vi "Is Homed.vi"(8 "error in (no error)":errorcluster, 11 "Gantry in":refnum<class "Gantry.lvclass">) -> (0 "error out":errorcluster, 2 "homed?":bool, 3 "Gantry out":refnum<class "Gantry.lvclass">)   [LabVIEW 2026, in "Gantry.lvclass"]
uses:
  Gantry.lvclass
  <instrlib>/Aerotech Automation1/Status/TypeDefs/Axis Status Items Cluster.ctl
  <instrlib>/Aerotech Automation1/Status/TypeDefs/Axis Status Item.ctl
  <instrlib>/Aerotech Automation1/Status/Wrappers/Add Axis Status Item.vi
  <instrlib>/Aerotech Automation1/Status/Wrappers/Read Axis Status Item.vi
  <instrlib>/Aerotech Automation1/Status/Status.lvlib
  <instrlib>/Aerotech Automation1/Aerotech Automation1.lvlib
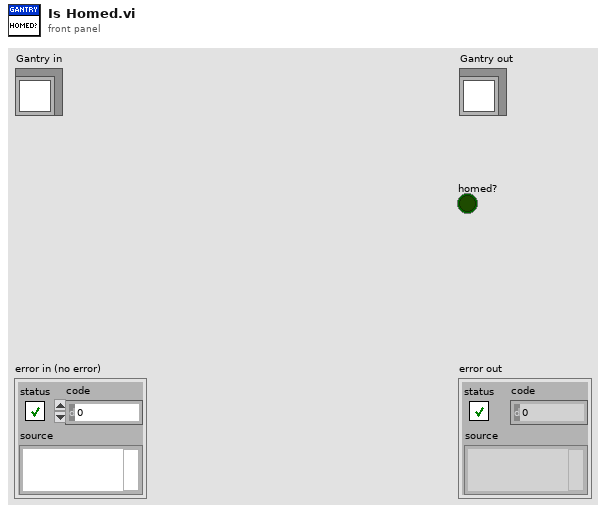
[diagram p1: front panel]
types:
  T1 = typedef "Virtual Modes.ctl" = enum16{"Nonvirtual", "Virtual"}
  T2 = typedef "ControllerDiagPacket.ctl" = cluster{"Number of Diag Packets":i32, "Axes":T3[], "error":errorcluster}
  T3 = typedef "AxisDiagPacket.ctl" = cluster{"Axis Name":string, "Analog Input 0":dbl, "Analog Input 1":dbl, "Axis Fault (num)":i32, "Axis Fault (str)":string, "Axis Fault (bits)":cluster{"AmplifierFault":bool, "AmplifierTemperatureFault":bool, "CcwEndOfTravelLimitFault":bool, "CcwSoftwareLimitFault":bool, "CommunicationLostFault":bool, "CwEndOfTravelLimitFault":bool, "CwSoftwareLimitFault":bool, "EmergencyStopFault":bool, "EncoderFault":bool, "ExternalFault":bool, "FeedbackScalingFault":bool, "GantryMisalignFault ":bool, "HallSensorFault":bool, "InPositionTimeoutFault":bool, "InternalFault":bool, "MarkerSearchFault":bool, "MaxVelocityCommandFault":bool, "MissedInterruptFault":bool, "MotorTemperatureFault":bool, "None":bool, "OverCurrentFault":bool, "PositionErrorFault":bool, "PositionFeedbackFault":bool, "PowerSupplyFault":bool, "ProbeInputFault":bool, "SafeZoneFault":bool, "VelocityErrorFault":bool, "VelocityFeedbackFault":bool, "VoltageClampFault":bool}, "Axis Status (num)":i32, "Axis Status (str)":string, "Axis Status (bits)":cluster{"BacklashActive":bool, "CalibrationEnabled1D":bool, "CalibrationEnabled2D":bool, "CommandValid":bool, "DriveAbortPending":bool, "DrivePending":bool, "Enabling":bool, "GainMappingEnabled":bool, "GantryAligned":bool, "GantryRealigning":bool, "Homed":bool, "Homing":bool, "IFOVEnabled":bool, "JogGenerating":bool, "Jogging":bool, "JoystickControl":bool, "MasterSlaveControl":bool, "MotionBlocked":bool, "MotionClamped":bool, "MoveDone":bool, "None":bool, "NotVirtual":bool, "Profiling":bool, "Stability0":bool, "Stability1":bool, "TrajectoryFiltering":bool, "WaitDone":bool}, "Current Command":sgl, "Current Error":sgl, "Current Feedback":sgl, "Digital Inputs":i32, "Digital Outputs":i32, "Drive Status":i32, "Drive Status (str)":string, "Drive Status (bits)":cluster{"AccelerationPhase":bool, "AutofocusActive":bool, "BrakeOutput":bool, "CcwEndOfTravelLimitInput":bool, "CosineEncoderError":bool, "CurrentClamp":bool, "CwEndOfTravelLimitInput":bool, "DecelerationPhase":bool, "DualLoopActive":bool, "EmergencyStopInput":bool, "Enabled":bool, "EncoderClipping":bool, "GalvoCalibrationEnabled":bool, "GalvoPowerCorrection":bool, "HallAInput":bool, "HallBInput":bool, "HallCInput":bool, "HighResolutionMode":bool, "HomeLimitInput":bool, "InPosition":bool, "InPosition2":bool, "MarkerInput":bool, "MarkerLatch":bool, "MoveActive":bool, "NoMotorSupply":bool, "None":bool, "PowerLimiting":bool, "ProgrammingFlash":bool, "ProgrammingMXH":bool, "PSOHaltLatch":bool, "ServoControl":bool, "SineEncoderError":bool}, "Position Feedback Auxiliary":dbl, "Position Command":dbl, "Position Error":dbl, "Position Feedback":dbl, "Program Position Command":dbl, "Program Position Error":dbl, "Program Position Feedback":dbl, "Velocity Command":dbl, "Velocity Error":dbl, "Velocity Feedback":dbl}
  T4 = typedef "Aerotech Automation1.lvlib/Status.lvlib/Axis Status Items Cluster.ctl" = cluster{"Axis Name":string, "axisStatusItem":T5}
  T5 = typedef "Aerotech Automation1.lvlib/Status.lvlib/Axis Status Item.ctl" = i32
  T6 = typedef "Aerotech Automation1.lvlib/Status.lvlib/Status Refnums.ctl" = cluster{"Status":refnum<k24>, "Status Config":refnum<k24>}
  T7 = typedef "Aerotech Automation1.lvlib/Status.lvlib/Axis Status Cluster.ctl" = cluster{"Homed":bool, "Profiling":bool, "WaitDone":bool, "CommandValid":bool, "Homing":bool, "Enabling":bool, "Unused 6":bool, "JogGenerating":bool, "Jogging":bool, "DrivePending":bool, "DriveAbortPending":bool, "TrajectoryFiltering":bool, "IfovEnabled":bool, "NotVirtual":bool, "CalibrationEnabled1D":bool, "CalibrationEnabled2D":bool, "CammingGearingControl":bool, "JoystickControl":bool, "BacklashActive":bool, "GainMappingEnabled":bool, "TransformationInput":bool, "TransformationOutput":bool, "MotionDone":bool, "MotionClamped":bool, "GantryAligned":bool, "GantryDriveControlRealigning":bool, "Unused 26":bool, "ThermoCompEnabled":bool, "Unused 28":bool, "Unused 29":bool, "Unused 30":bool, "Unused 31":bool}
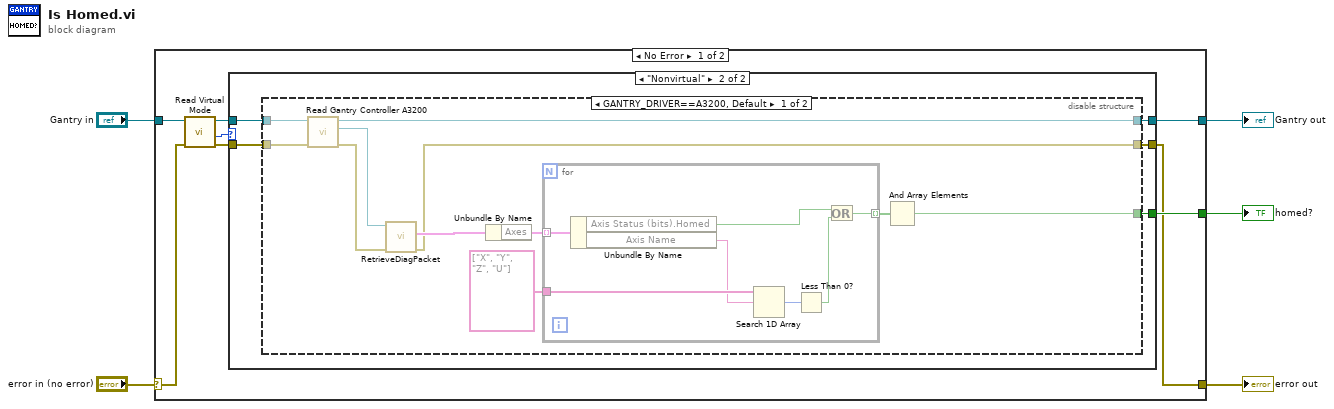
[diagram p0: block diagram]
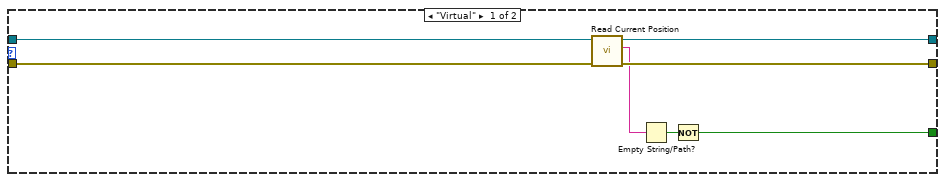
[diagram p2: hidden frame]
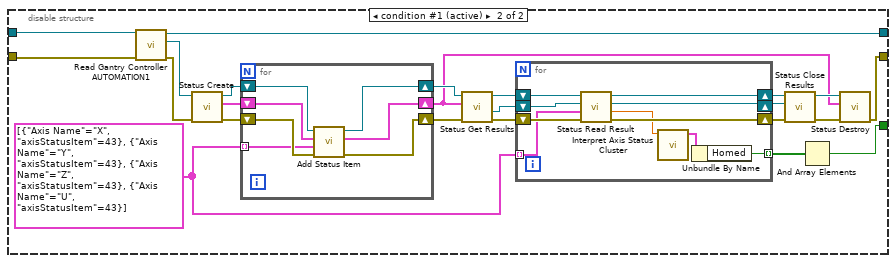
[diagram p3: hidden frame]
diagram:
  n1 = case shown="No Error" "error in (no error)" {
    selector: "error in (no error)" -> [w8 w85]
    tunnel: [w11 w85] -> w4
    tunnel: [w13 w84] -> w2
    tunnel: "Gantry in" -> [w10 w84]
    tunnel: [w12 _] -> w1
    frame No Error {
      n2 = call-dynamic "Read Virtual Mode.vi"("error in (no error)"=w8, "Gantry in"=w10) -> ("error out"=w7:errorcluster, "Virtual Mode"=w6:T1, "Gantry out"=w9:refnum<class "Gantry.lvclass">)  [unwired: 6 in, 1 out]
      n3 = case shown="\"Nonvirtual\"" w6 {
        tunnel: w9 -> [w20 w23]
        tunnel: [w18 w22] -> w13
        tunnel: w7 -> [w19 w21]
        tunnel: [w17 w24] -> w11
        tunnel: [w14 w25] -> w12
        frame "Virtual" {
          n4 = call-dynamic "Read Current Position.vi"("error in"=w19, "Gantry in"=w20) -> ("error out"=w17:errorcluster, "Current Position"=w16:string, "Gantry out"=w18:refnum<class "Gantry.lvclass">)  [unwired: 7 in]
          n5 = Empty String/Path?(string/path=w16) -> (empty?=w15:bool)
          n6 = Not(x=w15) -> (.not. x?=w14:bool)
        }
        frame "Nonvirtual" {
          n7 = disable-structure shown="GANTRY_DRIVER==A3200, Default" {
            disable-tunnel: [w32 w48] -> w25
            disable-tunnel: [w31 w47] -> w24
            disable-tunnel: w23 -> [w30 w46]
            disable-tunnel: [w29 w44] -> w22
            disable-tunnel: w21 -> [w28 w45]
            frame condition #0 {
              n8 = call "Read Gantry Controller A3200.vi"("error in (no error)"=w28, "Gantry in"=w30) -> ("error out"=w27:errorcluster, "A3200 controller out"=w26:refnum<k24>, "Gantry out"=w29:refnum<class "Gantry.lvclass">)  [unwired: 7 in]
              n9 = call "RetrieveDiagPacket.vi"("error in (no error)"=w27, "Controller In"=w26) -> ("error out"=w31:errorcluster, "ControllerDiagPacket"=w36:T2)  [unwired: 7 in, 1 out]
              n10 = Unbundle By Name(w36) -> ("Axes"=w35:T3[])
              n11 = for {
                tunnel: w35 -> [w43] mode=indexing
                tunnel: string[] ["X", "Y", "Z", "U"] -> [w42]
                tunnel: [w37] -> w33 mode=indexing
                n12 = Unbundle By Name(w43) -> ("Axis Status (bits).Homed"=w38:bool, "Axis Name"=w41:string)
                n13 = Search 1D Array(1D array=w42, element=w41) -> (index of element=w40:i32)  [unwired: 1 in]
                n14 = Less Than 0?(x=w40) -> (x < 0?=w39:bool)
                n15 = Or(x=w38, y=w39) -> (x .or. y?=w37:bool)
              }
              n16 = And Array Elements(Boolean array=w33) -> (logical AND=w32:bool)
            }
            frame condition #1 (active) {
              w59 = T4[] [{"Axis Name"="X", "axisStatusItem"=43}, {"Axis Name"="Y", "axisStatusItem"=43}, {"Axis Name"="Z", "axisStatusItem"=43}, {"Axis Name"="U", "axisStatusItem"=43}]
              n17 = call "Read Gantry Controller AUTOMATION1.vi"("error in (no error)"=w45, "Gantry in"=w46) -> ("error out"=w65:errorcluster, "Controller AUTOMATION1"=w66:refnum<k24>, "Gantry out"=w44:refnum<class "Gantry.lvclass">)  [unwired: 7 in]
              n18 = call <instrlib>:"Status Create.vi"("error in (no error)"=w65, "Controller Refnum"=w66) -> ("error out"=w64:errorcluster, "Status Refnums"=w63:T6, "Controller Refnum out"=w62:refnum<k24>)  [unwired: 7 in]
              n19 = for {
                shift-right: [w78] -> w60
                shift-left: w64 -> [w82]
                shift-right: [w79] -> w51
                shift-left: w63 -> [w80]
                tunnel: w59 -> [w81] mode=indexing
                shift-right: [w77] -> w61
                shift-left: w62 -> [w83]
                n20 = call-poly <instrlib>:"Add Status Item.vi"("error in"=w82, "Axis Status Item"=w81, "Status Refnums"=w80, "Controller Refnum"=w83) -> ("error out"=w78:errorcluster, "Status Refnums out"=w79:T6, "Controller Refnum out"=w77:refnum<k24>)  [unwired: 5 in]
              }
              n21 = call <instrlib>:"Status Get Results.vi"("error in (no error)"=w60, "Status Refnums"=w51, "Controller Refnum"=w61) -> ("error out"=w57:errorcluster, "GetStatusItems"=w56:refnum<k24>, "Controller Refnum out"=w58:refnum<k24>)  [unwired: 5 in, 1 out]
              n22 = for {
                tunnel: w59 -> [w73] mode=indexing
                shift-right: [w72] -> w55
                shift-left: w58 -> [w76]
                shift-right: [w74] -> w52
                shift-left: w57 -> [w75]
                shift-right: [w70] -> w53
                shift-left: w56 -> [w71]
                tunnel: [w67] -> w49 mode=indexing
                n23 = call-poly <instrlib>:"Status Read Result.vi"("error in (no error)"=w75, "Axis Status Item"=w73, "Status Results Refnum"=w71, "Controller Refnum"=w76) -> ("error out"=w74:errorcluster, "Data"=w69:dbl, "Status Results Refnum out"=w70:refnum<k24>, "Controller Refnum out"=w72:refnum<k24>)  [unwired: 4 in]
                n24 = call <instrlib>:"Interpret Axis Status Cluster.vi"("Data"=w69) -> ("Axis Status Cluster"=w68:T7)  [unwired: 10 in]
                n25 = Unbundle By Name(w68) -> ("Homed"=w67:bool)
              }
              n26 = call <instrlib>:"Status Close Results.vi"("error in (no error)"=w52, "Status Results Refnum"=w53, "Controller Refnum"=w55) -> ("error out"=w50:errorcluster, "Controller Refnum out"=w54:refnum<k24>)  [unwired: 7 in]
              n27 = And Array Elements(Boolean array=w49) -> (logical AND=w48:bool)
              n28 = call <instrlib>:"Status Destroy.vi"("error in"=w50, "Status Refnums"=w51, "Controller Refnum"=w54) -> ("error out"=w47:errorcluster)  [unwired: 7 in, 1 out]
            }
          }
        }
      }
    }
    frame Error {
    }
  }
  "error out" <- w4
  "Gantry out" <- w2
  "homed?" <- w1
